vi "_script_fix_Find Event Stucture Ref vi.vi"   [LabVIEW 2014]
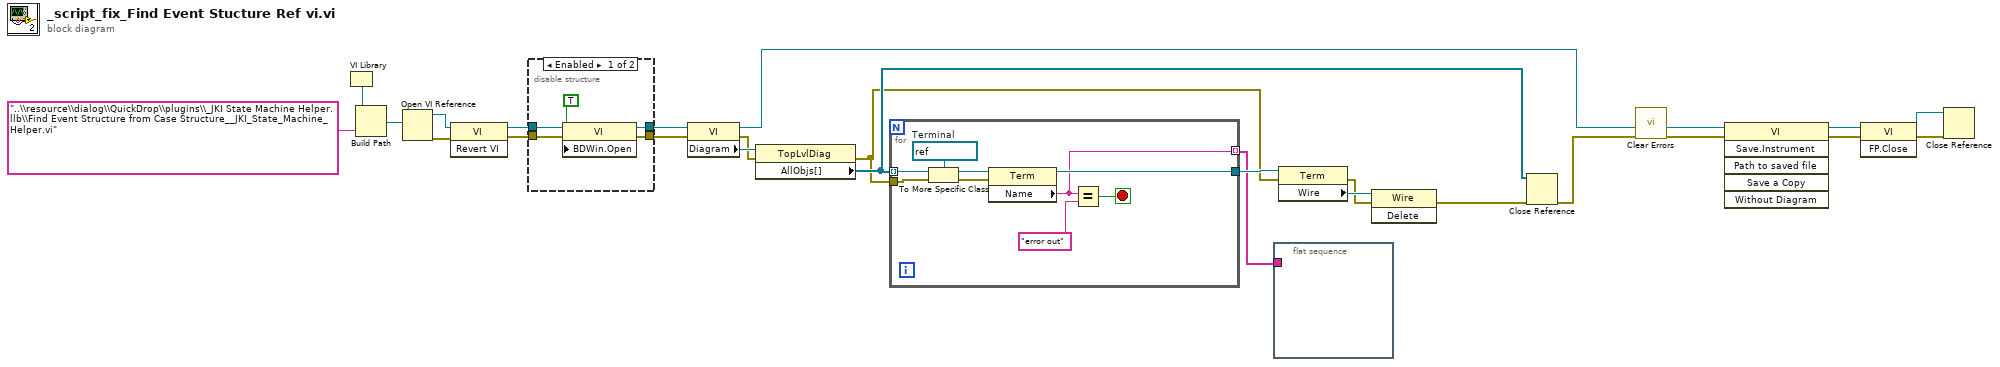
[diagram p0: block diagram]
diagram:
  n1 = VI Library() -> (path=w23:path)
  n2 = Build Path(base path=w23, name or relative path="..\\resource\\dialog\\QuickDrop\\plugins\\_JKI State Machine Helper.llb\\Find Event Structure from Case Structure__JKI_State_Machine_Helper.vi") -> (appended path=w21:path)
  n3 = Open VI Reference(vi path=w21) -> (vi reference=w24:refnum<vi>, error out=w25:errorcluster)  [unwired: 5 in]
  n4 = invoke class="VI" method="Revert VI"(reference=w24, error in=w25) -> (reference out=w20:refnum<vi>, error out=w19:errorcluster)  [unwired: 1 in, 1 out]
  n5 = disable-structure shown="Enabled" {
    disable-tunnel: w20 -> [w30 w32]
    disable-tunnel: w19 -> [w29 w31]
    disable-tunnel: [w28 w32] -> w18
    disable-tunnel: [w27 w31] -> w17
    frame Enabled {
      n6 = property class="VI"(reference=w30, error in=w29, "BDWin.Open"=TRUE ("Block Diagram Window:Open")) -> (reference out=w28:refnum<vi>, error out=w27:errorcluster)
    }
    frame Disabled {
    }
  }
  n7 = property class="VI"(reference=w18, error in=w17) -> (reference out=w11:refnum<vi>, error out=w15:errorcluster, "Diagram"=w16:refnum<vi>)
  n8 = property class="TopLvlDiag"(reference=w16, error in=w15) -> (error out=w7:errorcluster, "AllObjs[]"=w9:refnum<vi>[])  [unwired: 1 out]
  n9 = for {
    tunnel: w9 -> [w41] mode=indexing
    tunnel: [w36] -> w14
    tunnel: w7 -> [w35]
    tunnel: [w33] -> w6 mode=indexing
    stop <- w37 stop-if-true
    w39 = refnum<vi> refnum  # Terminal
    n10 = To More Specific Class(target class=w39, reference=w41, error in=w35) -> (specific class reference=w40:refnum<vi>, error out=w34:errorcluster)
    n11 = property class="Term"(reference=w40, error in=w34) -> (reference out=w36:refnum<vi>, "Name"=w33:string)  [unwired: 1 out]
    n12 = Equal?(x=w33, y="error out") -> (x = y?=w37:bool)
  }
  n13 = flat-sequence {
    tunnel: w6 -> [_]
    frame #0 {
    }
  }
  n14 = property class="Term"(reference=w14, error in=w7) -> (error out=w12:errorcluster, "Wire"=w13:refnum<vi>)  [unwired: 1 out]
  n15 = invoke class="Wire" method="Delete"(reference=w13, error in=w12) -> (error out=w8:errorcluster)  [unwired: 1 in, 2 out]
  n16 = Close Reference(reference=w9, error in (no error)=w8) -> (error out=w10:errorcluster)
  n17 = call <vilib>:"Clear Errors.vi"("error in (no error)"=w10) -> ("error out"=w1:errorcluster)  [unwired: 6 in]
  n18 = invoke class="VI" method="Save.Instrument"(reference=w11, error in=w1) -> (reference out=w4:refnum<vi>, error out=w5:errorcluster)  [unwired: 4 in, 4 out]
  n19 = invoke class="VI" method="FP.Close"(reference=w4, error in=w5) -> (reference out=w2:refnum<vi>, error out=w3:errorcluster)  [unwired: 1 in, 1 out]
  n20 = Close Reference(reference=w2, error in (no error)=w3) -> ()  [unwired: 1 out]
